vi "Autonomous Independent.vi"() -> ()   [LabVIEW 2016]
doc: "This VI is called when autonomous begins, and will automatically be terminated when autonomous ends. You can carry out timed or sensor driven robot movement independently without needing to return to the caller."
uses:
  <vilib>/Rock Robotics/Network Tables/NT Read Number.vi
  1_25_17/Action_type_def.ctl
  <vilib>/Rock Robotics/WPI/Solenoid/WPI_SolenoidValue.ctl
panel:
  in  "Value":T1=enum."Forward"
  out "Auto Mode":dbl=3.0
  in  "Auton_Modes":T3(array[cluster])=[{"Actions"=[{"Action"=enum."Drive", "Effort"=0.55, "Duration"=3.5}, {"Action"=enum."Nothing", "Effort"=0.0, "Duration"=0.0}]}, {"Actions"=[{"Action"=enum."Art Down", "Effort"=0.0, "Duration"=1.0}, {"Action"=enum."Drive", "Effort"=0.75, "Duration"=5.0}, {"Action"=enum."Art Up", "Effort"=0.0, "Duration"=1.0}]}, {"Actions"=[{"Action"=enum."Drive", "Effort"=1.0, "Duration"=3.0}, {"Action"=enum."Art Down", "Effort"=0.0, "Duration"=1.0}, {"Action"=enum."Drive", "Effort"=0.75, "Duration"=3.5}, {"Action"=enum."Art Up", "Effort"=0.0, "Duration"=1.0}]}, {"Actions"=[{"Action"=enum."Art Down", "Effort"=0.0, "Duration"=0.5}, {"Action"=enum."Drive", "Effort"=0.8, "Duration"=5.28}, {"Action"=enum."Art Up", "Effort"=0.0, "Duration"=1.0}, {"Action"=enum."Turn", "Effort"=-0.8, "Duration"=1.8}, {"Action"=enum."Nothing", "Effort"=0.0, "Duration"=0.1}, {"Action"=enum."Drive", "Effort"=0.8, "Duration"=1.75}, {"Action"=enum."Art Down", "Effort"=0.0, "Duration"=0.5}, {"Action"=enum."climb", "Effort"=0.0, "Duration"=4.0}]}, {"Actions"=[{"Action"=enum."Shift", "Effort"=0.0, "Duration"=0.0}, {"Action"=enum."Drive", "Effort"=1.0, "Duration"=0.1}, {"Action"=enum."Nothing", "Effort"=0.0, "Duration"=0.1}, {"Action"=enum."Drive", "Effort"=1.0, "Duration"=3.0}]}, {"Actions"=[{"Action"=enum."Shift", "Effort"=0.0, "Duration"=0.0}, {"Action"=enum."Drive", "Effort"=1.0, "Duration"=0.1}, {"Action"=enum."Nothing", "Effort"=0.0, "Duration"=0.1}, {"Action"=enum."Drive", "Effort"=1.0, "Duration"=3.0}]}, {"Actions"=[{"Action"=enum."Drive", "Effort"=0.55, "Duration"=4.0}, {"Action"=enum."Art Down", "Effort"=0.0, "Duration"=1.0}, {"Action"=enum."Drive", "Effort"=-0.5, "Duration"=0.6}, {"Action"=enum."Drive", "Effort"=0.75, "Duration"=1.0}, {"Action"=enum."Art Up", "Effort"=0.0, "Duration"=1.0}, {"Action"=enum."Drive", "Effort"=0.75, "Duration"=3.0}]}, {"Actions"=[{"Action"=enum."Art Down", "Effort"=0.0, "Duration"=0.5}, {"Action"=enum."Drive", "Effort"=0.55, "Duration"=4.25}, {"Action"=enum."Art Up", "Effort"=0.0, "Duration"=0.0}, {"Action"=enum."Nothing", "Effort"=0.0, "Duration"=0.3}, {"Action"=enum."Drive", "Effort"=0.9, "Duration"=2.0}]}, {"Actions"=[{"Action"=enum."Nothing", "Effort"=0.0, "Duration"=0.0}]}]
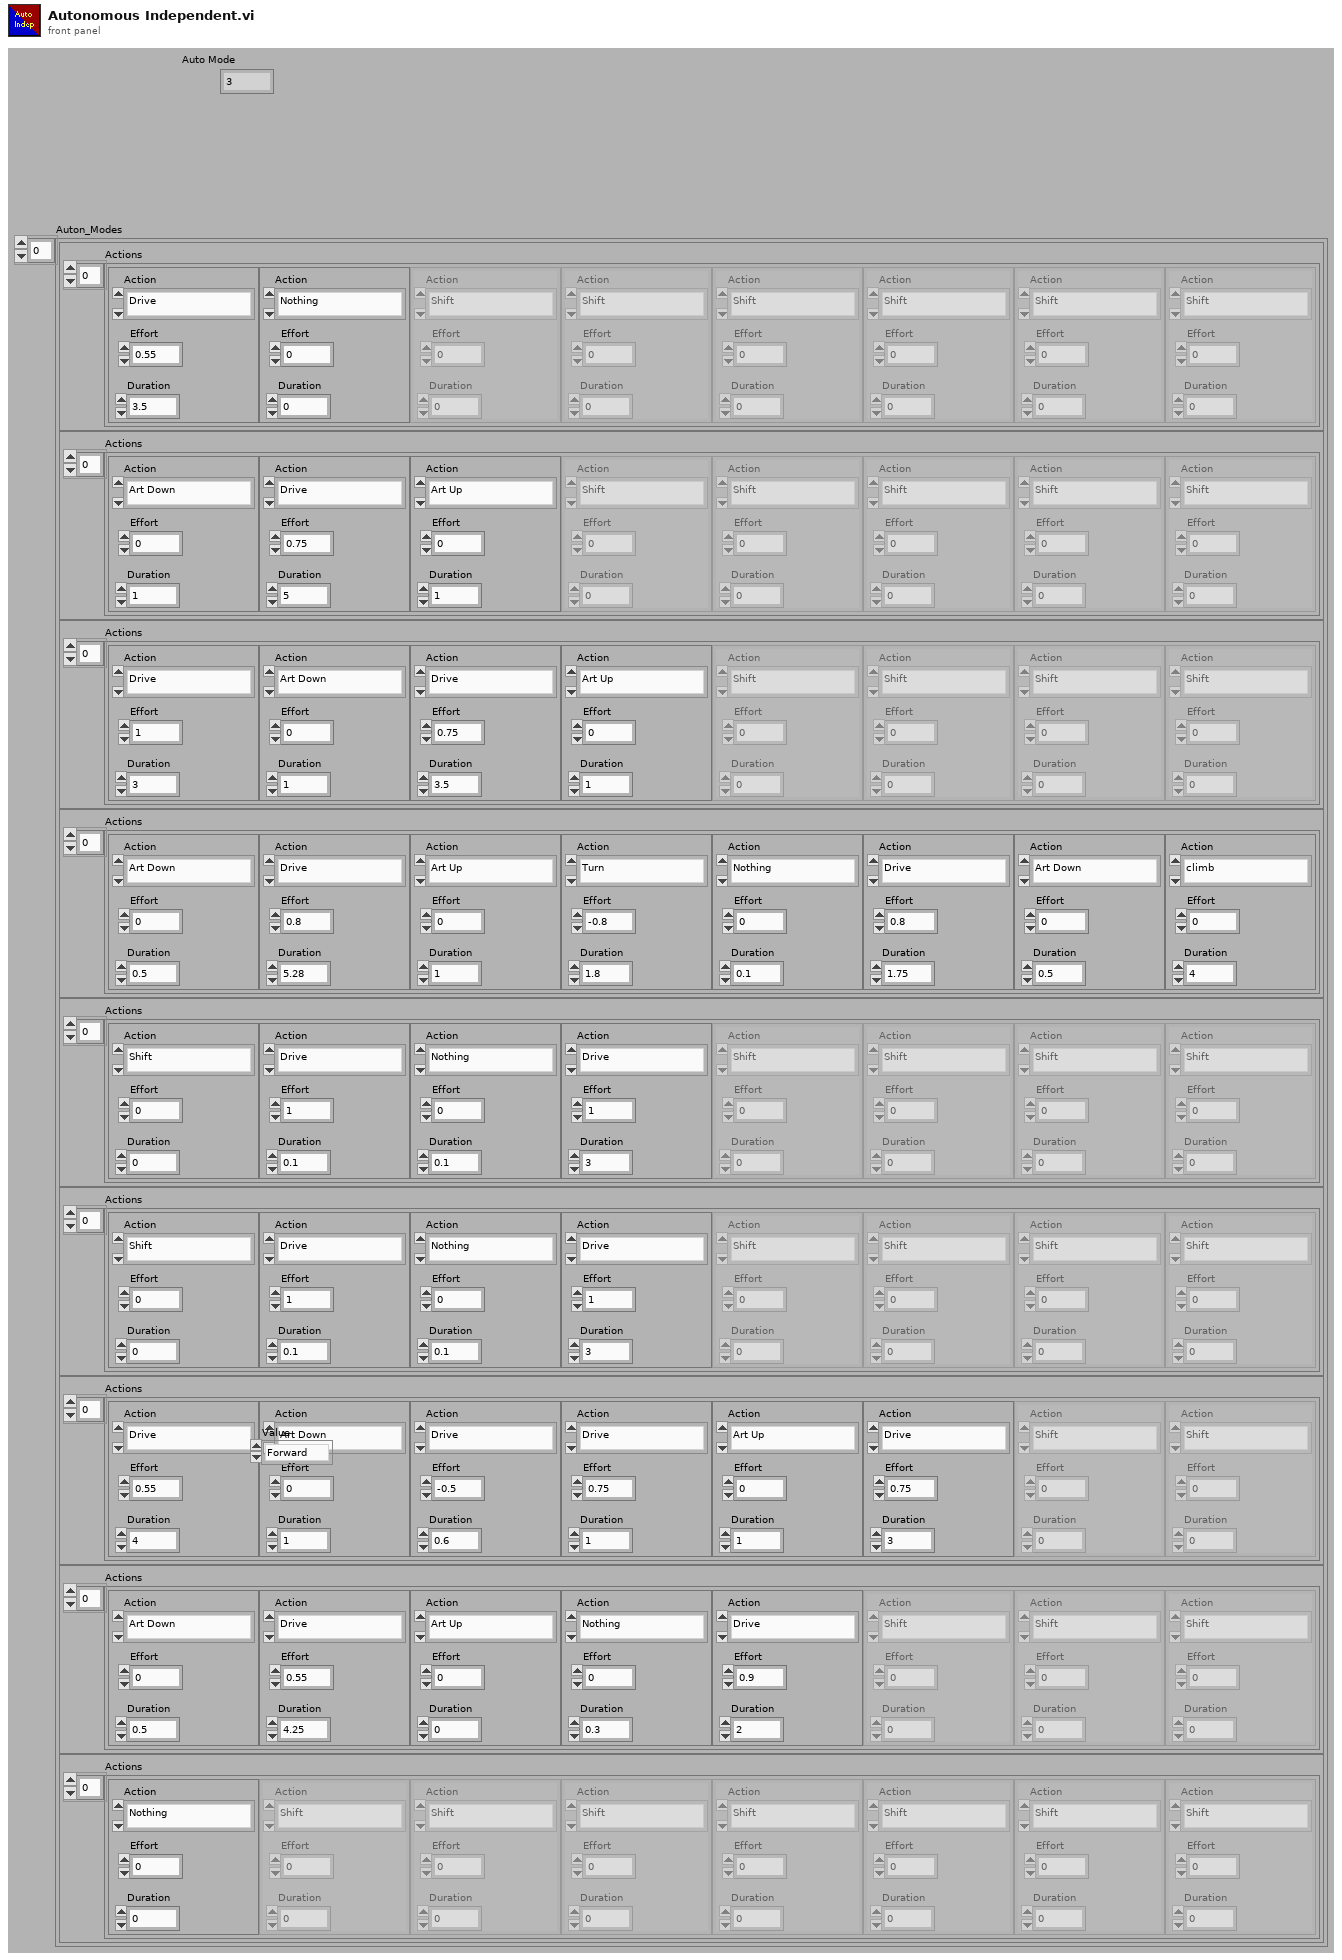
[diagram p1: front panel]
types:
  T1 = typedef "WPI_SolenoidValue.ctl" = enum16{"Off", "On", "Forward", "Reverse"}
  T2 = typedef "Action_type_def.ctl" = enum16{"Shift", "Shoot", "Move Articulates", "Nothing", "Drive", "Turn", "climb", "Art Up", "Art Down", "Test"}
  T3 = cluster{"Actions":cluster{"Action":T2, "Effort":dbl, "Duration":dbl}[]}[]
  T4 = cluster{"Actions":cluster{"Action":T2, "Effort":dbl, "Duration":dbl}[]}
  T5 = cluster{"Action":T2, "Effort":dbl, "Duration":dbl}[]
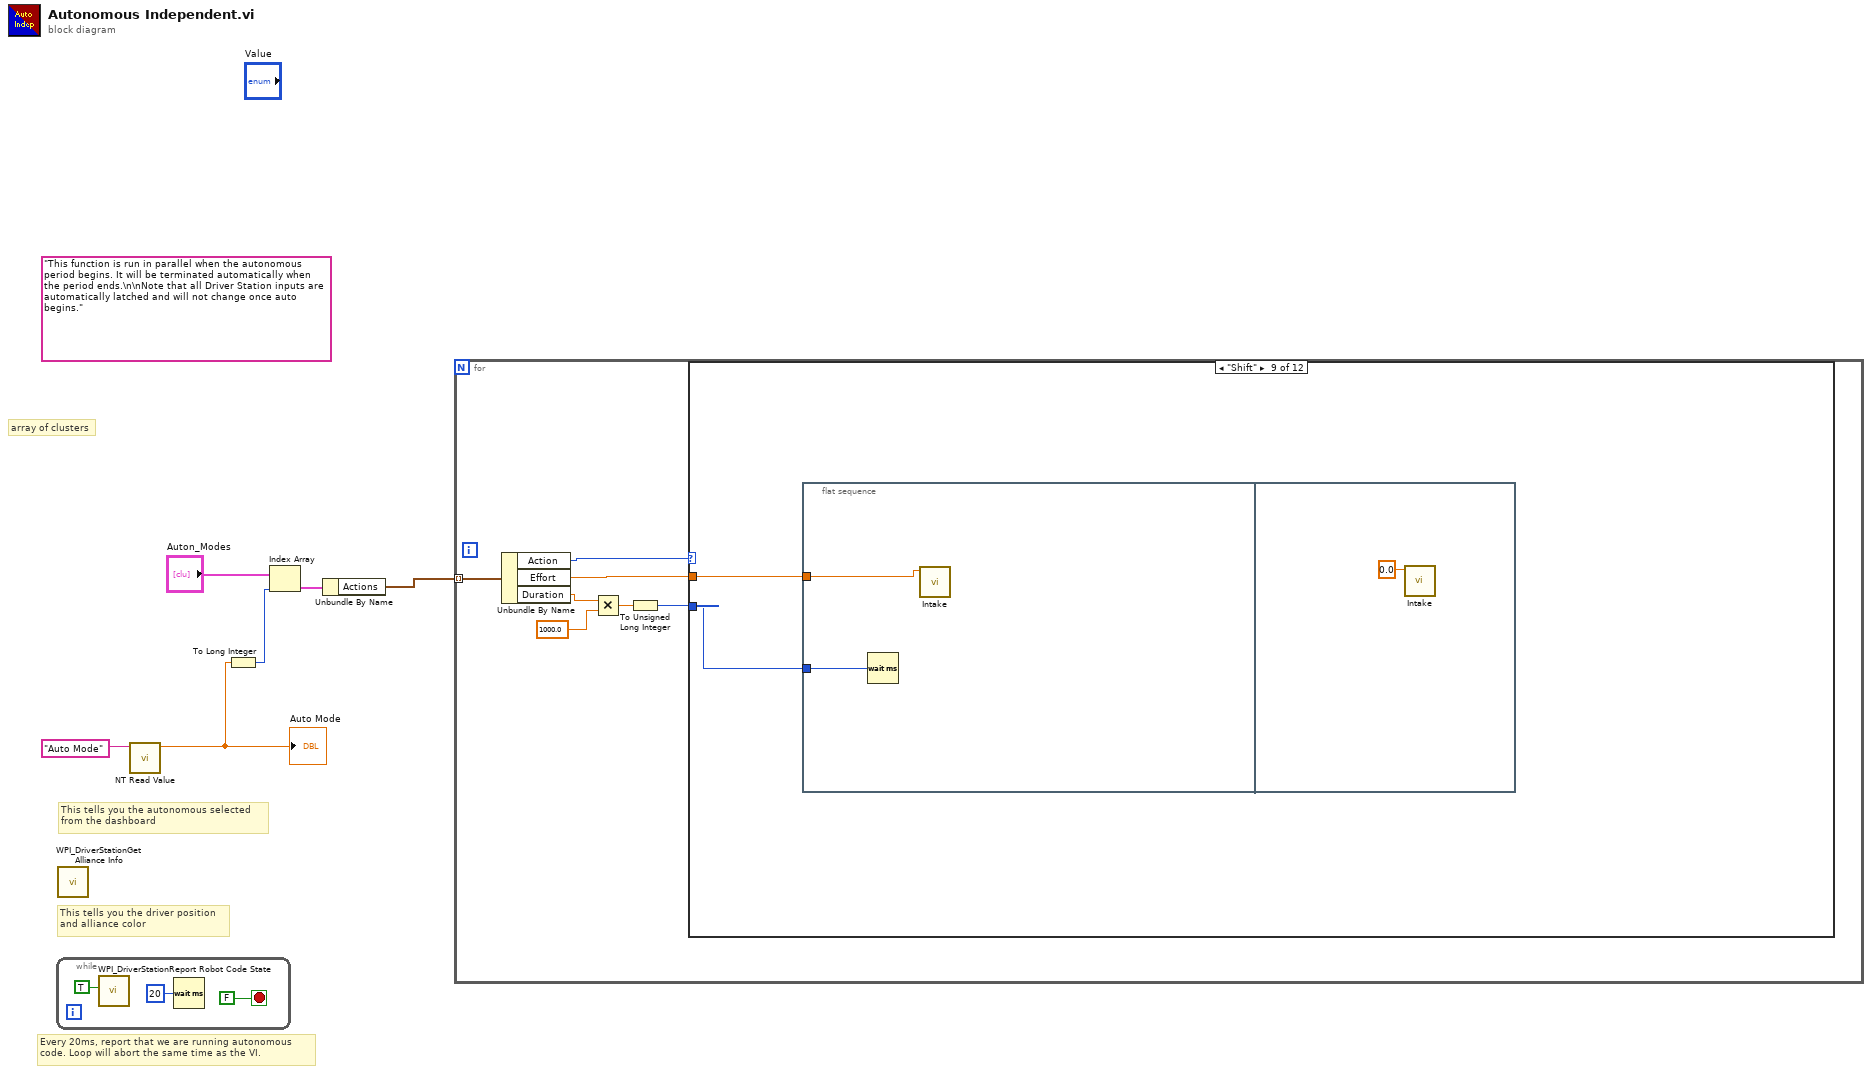
[diagram p0: block diagram]
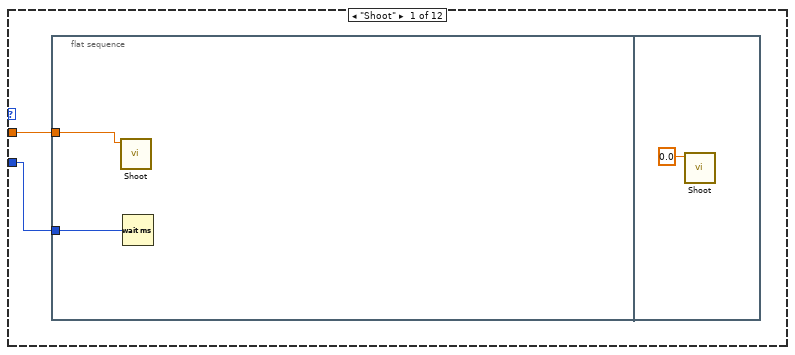
[diagram p2: hidden frame]
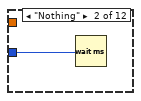
[diagram p3: hidden frame]
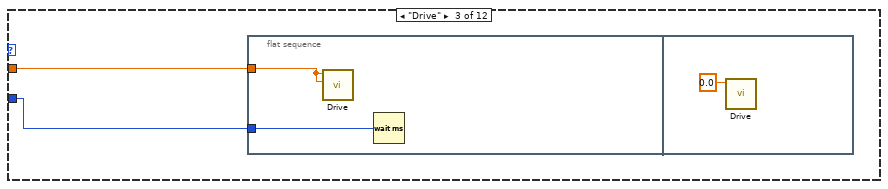
[diagram p4: hidden frame]
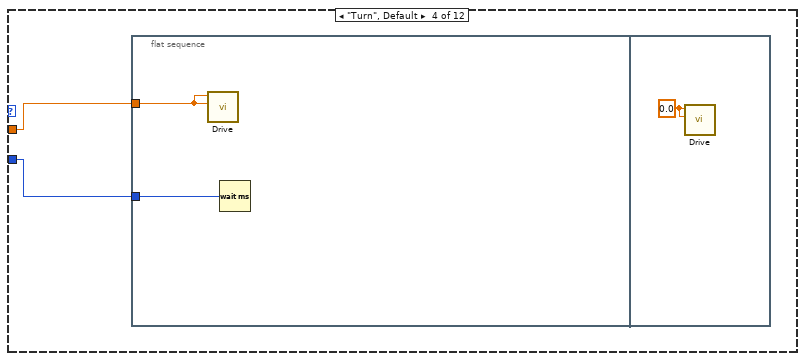
[diagram p5: hidden frame]
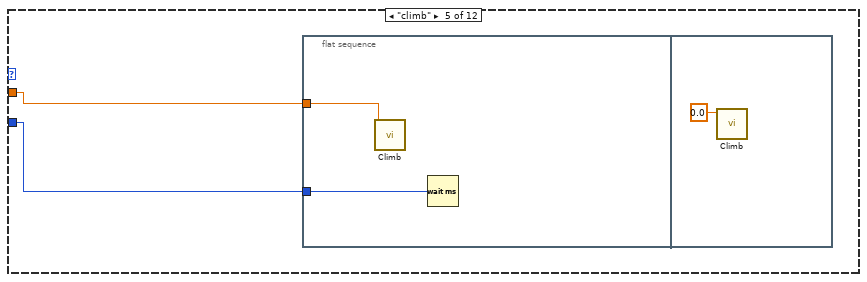
[diagram p6: hidden frame]
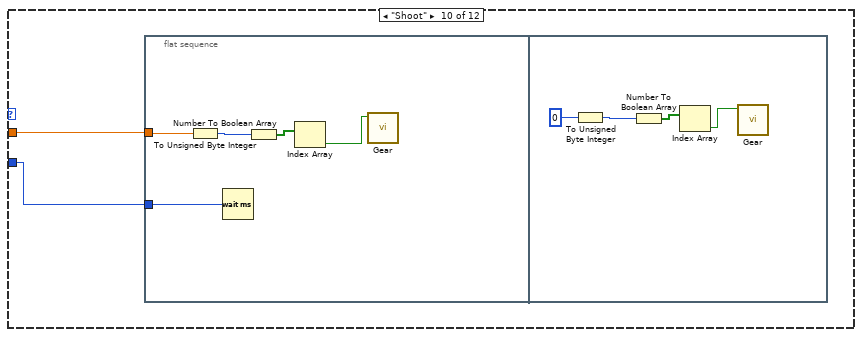
[diagram p10: hidden frame]
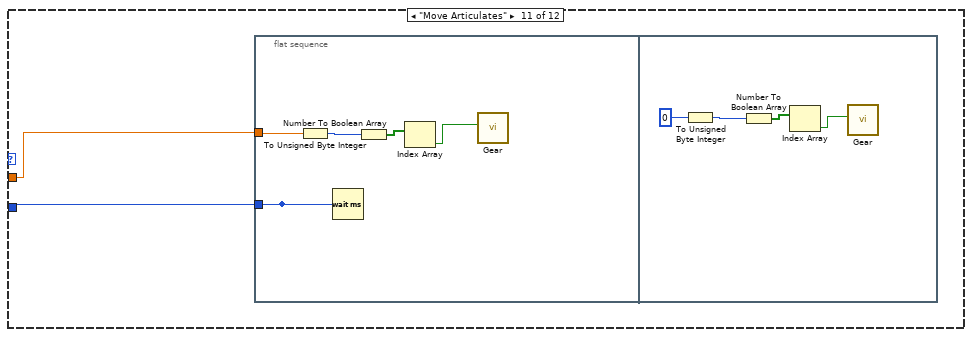
[diagram p11: hidden frame]
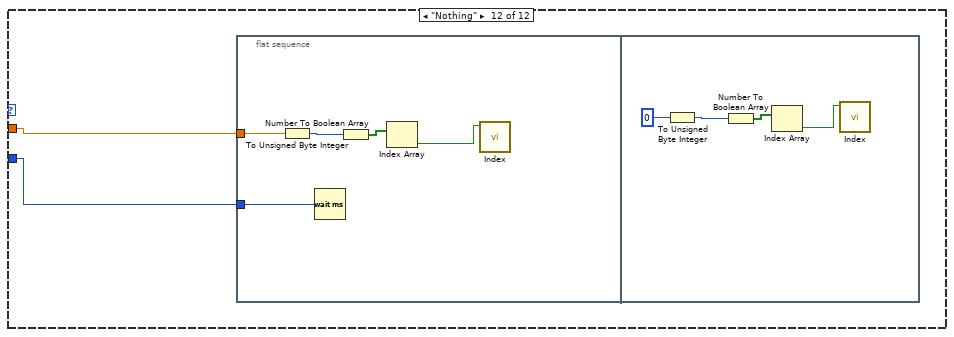
[diagram p12: hidden frame]
diagram:
  (unwired) "This function is run in parallel when the autonomous period begins. It will be terminated automatically when the period ends.\n\nNote that all Driver Station inputs are automatically latched and will not change once auto begins."
  # "This tells you the autonomous selected\nfrom the dashboard"
  # "array of clusters"
  # "Every 20ms, report that we are running autonomous\ncode. Loop will abort the same time as the VI."
  # "This tells you the driver position\nand alliance color"
  n1 = while {
    stop <- FALSE stop-if-true
    n2 = call <vilib>:"WPI_DriverStationReport Robot Code State.vi"("Autonomous"=TRUE) -> ()  [unwired: 10 in, 1 out]
    n3 = Wait (ms)(milliseconds to wait=u32 20) -> ()  [unwired: 1 out]
  }
  n4 = call <vilib>:"WPI_DriverStationGet Alliance Info.vi"() -> ()  [unwired: 12 out]
  n5 = call-poly <vilib>:"NT Read Value.vi"("Name"="Auto Mode") -> ("Numeric"=w1:dbl)  [unwired: 9 in, 1 out]
  "Auto Mode" <- w1
  n6 = To Long Integer(number=w1) -> (32bit integer=w3:i32)
  n7 = Index Array(array="Auton_Modes", index=w3) -> (element=w5:T4)
  n8 = Unbundle By Name(w5) -> ("Actions"=w6:T5)
  n9 = for {
    tunnel: w6 -> [w16] mode=indexing
    n10 = Unbundle By Name(w16) -> ("Action"=w15:T2, "Effort"=w14:dbl, "Duration"=w13:dbl)
    n11 = Multiply(x=w13, y=1000.0) -> (x*y=w11:dbl)
    n12 = To Unsigned Long Integer(number=w11) -> (unsigned 32bit integer=w10:u32)
    n13 = case shown="\" Intake\"" w15 {
      tunnel: w14 -> [w18 _ w24 w29 w34 _ _ _ w39 w43 w55 w65]
      tunnel: w10 -> [w17 w22 w23 w28 w33 _ _ _ w38 w44 w54 w66]
      frame "Shoot" {
        n14 = flat-sequence {
          tunnel: w18 -> [w20]
          tunnel: w17 -> [w19]
          frame #0 {
            n15 = call "Shoot.vi"("Effort"=w20) -> ()  [unwired: 11 in]
            n16 = Wait (ms)(milliseconds to wait=w19) -> ()  [unwired: 1 out]
          }
          frame #1 {
            n17 = call "Shoot.vi"("Effort"=0.0) -> ()  [unwired: 11 in]
          }
        }
      }
      frame "Nothing" {
        n18 = Wait (ms)(milliseconds to wait=w22) -> ()  [unwired: 1 out]
      }
      frame "Drive" {
        n19 = flat-sequence {
          tunnel: w24 -> [w26]
          tunnel: w23 -> [w25]
          frame #0 {
            n20 = call "Drive.vi"("Drive R"=w26, "Drive L"=w26) -> ()  [unwired: 10 in]
            n21 = Wait (ms)(milliseconds to wait=w25) -> ()  [unwired: 1 out]
          }
          frame #1 {
            n22 = call "Drive.vi"("Drive L"=0.0) -> ()  [unwired: 11 in]
          }
        }
      }
      frame "Turn", Default {
        n23 = flat-sequence {
          tunnel: w29 -> [w31]
          tunnel: w28 -> [w30]
          frame #0 {
            n24 = call "Drive.vi"("Drive R"=w31, "Drive L"=w31) -> ()  [unwired: 10 in]
            n25 = Wait (ms)(milliseconds to wait=w30) -> ()  [unwired: 1 out]
          }
          frame #1 {
            w32 = 0.0 ("Drive L")
            n26 = call "Drive.vi"("Drive R"=w32, "Drive L"=w32) -> ()  [unwired: 10 in]
          }
        }
      }
      frame "climb" {
        n27 = flat-sequence {
          tunnel: w34 -> [w36]
          tunnel: w33 -> [w35]
          frame #0 {
            n28 = call "Climb.vi"("Effort"=w36) -> ()  [unwired: 11 in]
            n29 = Wait (ms)(milliseconds to wait=w35) -> ()  [unwired: 1 out]
          }
          frame #1 {
            n30 = call "Climb.vi"("Effort"=0.0) -> ()  [unwired: 11 in]
          }
        }
      }
      frame "Art Up" {
      }
      frame "Art Down" {
      }
      frame "Test" {
      }
      frame "Shift" {
        n31 = flat-sequence {
          tunnel: w39 -> [w41]
          tunnel: w38 -> [w40]
          frame #0 {
            n32 = Wait (ms)(milliseconds to wait=w40) -> ()  [unwired: 1 out]
            n33 = call "Intake.vi"("Effort"=w41) -> ()  [unwired: 11 in]
          }
          frame #1 {
            n34 = call "Intake.vi"("Effort"=0.0) -> ()  [unwired: 11 in]
          }
        }
      }
      frame "Shoot" {
        n35 = flat-sequence {
          tunnel: w44 -> [w49]
          tunnel: w43 -> [w48]
          frame #0 {
            n36 = To Unsigned Byte Integer(number=w48) -> (unsigned 8bit integer=w47:u8)
            n37 = Wait (ms)(milliseconds to wait=w49) -> ()  [unwired: 1 out]
            n38 = Number To Boolean Array(number=w47) -> (Boolean array=w46:bool[])
            n39 = Index Array(array=w46) -> (element=w45:bool)  [unwired: 1 in]
            n40 = call "Gear.vi"("Gear0?"=w45) -> ()  [unwired: 11 in]
          }
          frame #1 {
            n41 = To Unsigned Byte Integer(number=u8 0) -> (unsigned 8bit integer=w52:u8)
            n42 = Number To Boolean Array(number=w52) -> (Boolean array=w53:bool[])
            n43 = Index Array(array=w53) -> (element=w50:bool)  [unwired: 1 in]
            n44 = call "Gear.vi"("Gear0?"=w50) -> ()  [unwired: 11 in]
          }
        }
      }
      frame "Move Articulates" {
        n45 = flat-sequence {
          tunnel: [w56] -> _
          tunnel: w55 -> [w60]
          tunnel: w54 -> [w56]
          frame #0 {
            n46 = To Unsigned Byte Integer(number=w60) -> (unsigned 8bit integer=w59:u8)
            n47 = Wait (ms)(milliseconds to wait=w56) -> ()  [unwired: 1 out]
            n48 = Number To Boolean Array(number=w59) -> (Boolean array=w58:bool[])
            n49 = Index Array(array=w58) -> (element=w57:bool)  [unwired: 1 in]
            n50 = call "Gear.vi"("Gear1?"=w57) -> ()  [unwired: 11 in]
          }
          frame #1 {
            n51 = To Unsigned Byte Integer(number=u8 0) -> (unsigned 8bit integer=w63:u8)
            n52 = Number To Boolean Array(number=w63) -> (Boolean array=w64:bool[])
            n53 = Index Array(array=w64) -> (element=w61:bool)  [unwired: 1 in]
            n54 = call "Gear.vi"("Gear1?"=w61) -> ()  [unwired: 11 in]
          }
        }
      }
      frame "Nothing" {
        n55 = flat-sequence {
          tunnel: w66 -> [w68]
          tunnel: w65 -> [w67]
          frame #0 {
            n56 = To Unsigned Byte Integer(number=w67) -> (unsigned 8bit integer=w71:u8)
            n57 = Wait (ms)(milliseconds to wait=w68) -> ()  [unwired: 1 out]
            n58 = Number To Boolean Array(number=w71) -> (Boolean array=w70:bool[])
            n59 = Index Array(array=w70) -> (element=w69:bool)  [unwired: 1 in]
            n60 = call "Index.vi"("Index?"=w69) -> ()  [unwired: 11 in]
          }
          frame #1 {
            n61 = To Unsigned Byte Integer(number=u8 0) -> (unsigned 8bit integer=w74:u8)
            n62 = Number To Boolean Array(number=w74) -> (Boolean array=w75:bool[])
            n63 = Index Array(array=w75) -> (element=w72:bool)  [unwired: 1 in]
            n64 = call "Index.vi"("Index?"=w72) -> ()  [unwired: 11 in]
          }
        }
      }
    }
  }
